vi "HandleItemActivation.vi"(8 "error in (no error)":errorcluster, 11 "GettingStartedWindow.lvlib:ProjectWizard.lvclass":refnum<class "ProjectWizard.lvclass">) -> (0 "error out":errorcluster, 3 "GettingStartedWindow.lvlib:ProjectWizard.lvclass 2":refnum<class "ProjectWizard.lvclass">)   [LabVIEW 2009, in "NavScreen.lvlib" / "ProjectWizard.lvclass"]
uses:
  ProjectWizard.lvclass
panel:
  in  "message":string="Project wizards not really launched for this example."
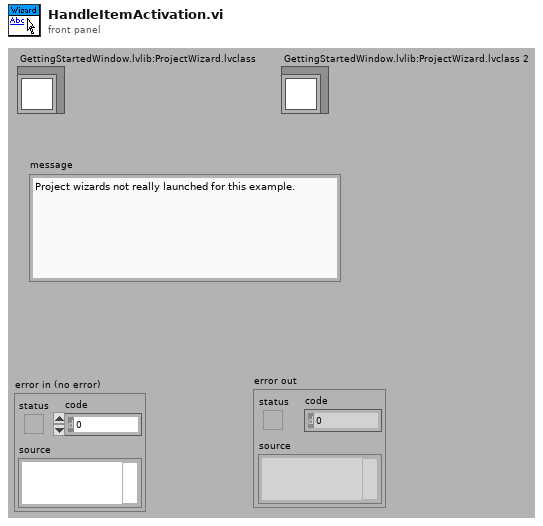
[diagram p1: front panel]
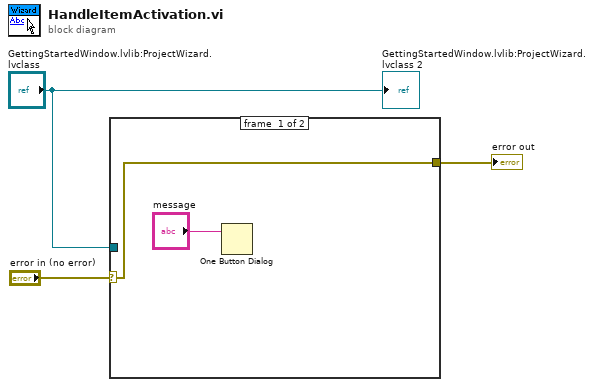
[diagram p0: block diagram]
diagram:
  n1 = case shown="No Error" "error in (no error)" {
    selector: "error in (no error)" -> [w4 w6]
    tunnel: [w4 w6] -> w2
    tunnel: "GettingStartedWindow.lvlib:ProjectWizard.lvclass" -> [_ _]
    frame #0 {
      n2 = One Button Dialog(message="message") -> ()  [unwired: 1 in, 1 out]
    }
    frame #1 {
    }
  }
  "error out" <- w2
  "GettingStartedWindow.lvlib:ProjectWizard.lvclass 2" <- "GettingStartedWindow.lvlib:ProjectWizard.lvclass"
